vi "FFT_DAS Acq USB-Thermocouple.vi"(11 "Temp Channel":refnum<k21>) -> ()   [LabVIEW 2010]
doc: "I. Description:\nThis example demonstrates how to make temperature measurement using a thermocouple.\n\nII. Instructions for Running:\n1. Specify the Physical Channel where you have connected the thermocouple.\n2. Enter the Minimum and Maximum temperature values you expect to measure in degrees C. A smaller range will allow a more accurate measurement.\n3. Specify the type of thermocouple you are using.\n4. Thermocouple measurements require cold-junction compensation (CJC) to correctly scale them. Specify the source of your cold-junction compensation.\n5. If your CJC source is \"Internal\", skip the rest of steps.\n6. If your CJC source is \"Constant Value\", specify the value (usually room temperature) in degrees C.\n7. If your CJC source is \"Channel\", specify the CJC Channel name. \n\nIII. Block Diagram Steps:\n1. Create a Thermocouple (TC) temperature measurement channel.\n2. Call the Read VI to read one point of data.\n3. Call the Clear Task VI to clear the Task \n4. Use the popup dialog box to display an error if any.\n\nIV. I/O Connections Overview:\nConnect your thermocouple to the terminals corresponding to the Physical Channel I/O Control value."
uses:
  <vilib>/Utility/error.llb/DialogType.ctl
  <vilib>/Platform/TimedLoop/XDataNode/XDataNode.xnode
  <vilib>/Platform/TimedLoop/XDataNode/timing_clust.ctl
  <vilib>/Platform/TimedLoop/XDataNode/nitl_modes.ctl
  <vilib>/Platform/TimedLoop/XDataNode/wakeup.ctl
  <vilib>/DAQmx/read.llb/DAQmx Read (Analog DBL 1Chan 1Samp).vi
  <vilib>/daqmx/miscellaneous.llb/DAQmx Fill In Error Info.vi
  <vilib>/Platform/TimedLoop/XDataNode/XDNodeRunTimeDep.lvlib
panel:
  out "mSec":u32
  out "Loops":i32
  in  "stop":bool
  out "Measurement":cluster{"data":dbl, u32}(graph)
  out "Temperature":dbl(slide)=97.41100323624595 scale=0.0..100.0
  # "For instructions, select Help>>Show Context Help"
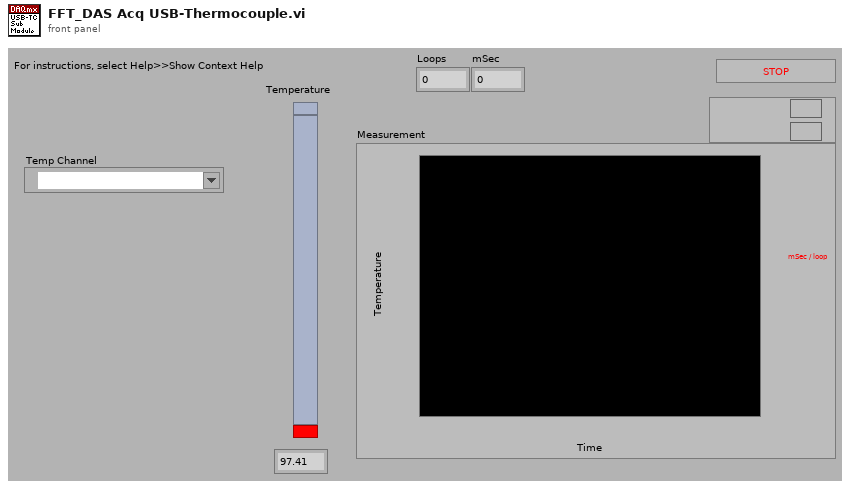
[diagram p1: front panel]
types:
  T1 = typedef "DialogType.ctl" = u16
  T2 = typedef "XDNodeRunTimeDep.lvlib/timing_clust.ctl" = cluster{"Expected End [f-1]":u64, "Actual End [f-1]":u64, "Finished Late? [f-1]":bool, "Expected End [i-1]":u64, "Actual End [i-1]":u64, "Finished Late? [i-1]":bool, "Expected Start [i]":u64, "Actual Start [i]":u64, "Expected Start [f]":u64, "Actual Start [f]":u64, "Source Name":string, "Structure Name":string, "Period":i64, "Deadline":i64, "Offset":i64, "Start":i64, "Priority":i32, "Timeout":i32, "Mode":T3, "Wakeup Reason":T4, "Error":errorcluster, "Source Type":string, "Secondary Source Type":string, "Global End Time":u64, "Global Start Time":u64, "Frame Duration":u64, "Iteration Duration":u64, "Assigned CPU":i32, "I/O Scan Engine Mode":u32}
  T3 = typedef "XDNodeRunTimeDep.lvlib/nitl_modes.ctl" = enum32{"No Change", "Process missed periods, maintain original phase", "Discard missed periods, maintain original phase", "Process missed periods, ignore original phase", "Discard missed periods, ignore original phase"}
  T4 = typedef "XDNodeRunTimeDep.lvlib/wakeup.ctl" = enum32{"Normal", "Aborted", "Asynchronous wakeup", "Timing source error", "Timed loop error", "Timeout"}
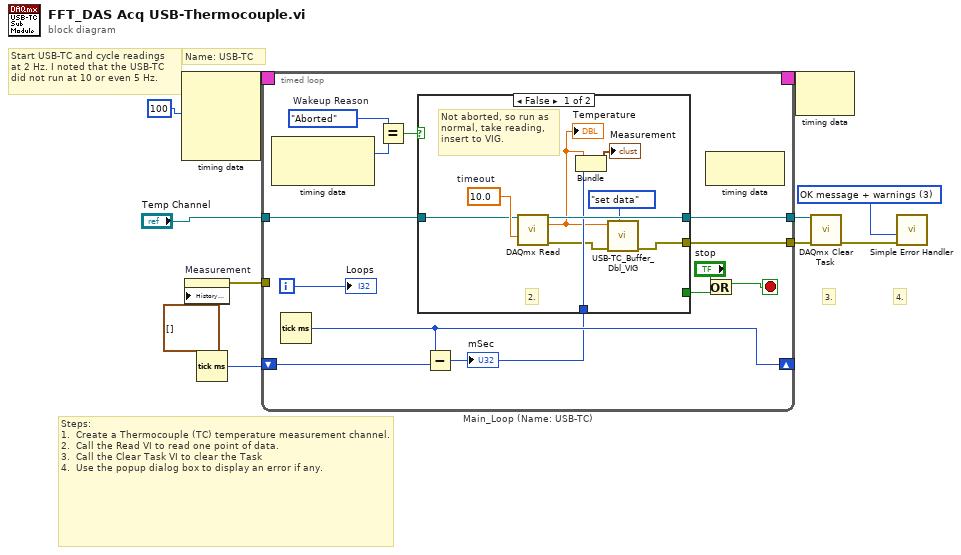
[diagram p0: block diagram]
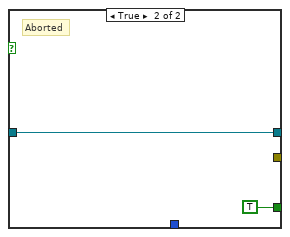
[diagram p2: hidden frame]
diagram:
  w11 = T1 3 items=["no dialog", "OK message", "continue or stop message", "OK message + warnings", "continue/stop + warnings"] ("type of dialog (OK msg:1)")
  # "Start USB-TC and cycle readings\nat 2 Hz. I noted that the USB-TC\ndid not run at 10 or even 5 Hz."
  # "Name: USB-TC"
  # "3."
  # "4."
  # "Steps: \n1.  Create a Thermocouple (TC) temperature measurement channel.\n2.  Call the Read VI to read one point of data.\n3.  Call the Clear Task VI to clear the Task  \n4.  Use the popup dialog box to display an error if any."
  n1 = node-c288(i64 100 ("Period")) -> (w7:T2)  [unwired: 3 in]
  n2 = property on="Measurement" class="WFChart (strict)"("History Data"=cluster{"data":dbl, u32}[] []) -> (error out=w4:errorcluster)  [unwired: 2 in, 1 out]
  n3 = Tick Count (ms)() -> (millisecond timer value=w3:u32)
  n4 = timed-loop "Main_Loop (Name: USB-TC)" {
    timing: w7 -> [_]
    timing-out: [_] -> w6
    tunnel: [w24] -> w10
    tunnel: [w23] -> w9
    tunnel: w4 -> [_]
    shift-right: [w19] -> _
    shift-left: w3 -> [w20]
    tunnel: "Temp Channel" -> [w12]
    i -> [w21]
    stop <- w14 stop-if-true
    w16 = wakeup."Aborted"  # Wakeup Reason
    n5 = node-c288() -> (w17:T4)  [unwired: 1 in, 1 out]
    n6 = Tick Count (ms)() -> (millisecond timer value=w19:u32)
    n7 = Equal?(x=w16, y=w17) -> (x = y?=w15:bool)
    n8 = Subtract(x=w19, y=w20) -> (x-y=w18:u32)
    "mSec" <- w18
    n9 = case shown="False" w15 {
      tunnel: [w32 w34] -> w24
      tunnel: [w27 _] -> w23
      tunnel: w18 -> [w31 _]
      tunnel: [_ TRUE] -> w13
      tunnel: w12 -> [w25 w34]
      frame False {
        w33 = 10.0  # timeout
        # "Not aborted, so run as\nnormal, take reading,\ninsert to VIG."
        # "2."
        n10 = call-poly <vilib>:"DAQmx Read.vi"("task/channels in"=w25, "timeout"=w33) -> ("task out"=w32:refnum<k21>, "data"=w29:dbl, "error out"=w28:errorcluster)  [unwired: 11 in]
        "Temperature" <- w29
        n11 = Bundle("data"=w29, w31) -> (→"Measurement":cluster{"data":dbl, u32})  [unwired: 1 in]
        n12 = call "USB-TC_Buffer_Dbl_VIG.vi"("Operation"=enum16{"get data", "set data", "initialize"}."set data", "error in"=w28, "Numeric"=w29) -> ("error out"=w27:errorcluster)  [unwired: 7 in, 1 out]
      }
      frame True {
        # "Aborted"
      }
    }
    n13 = node-c288() -> ()  [unwired: 1 in, 1 out]
    n14 = Or(x="stop", y=w13) -> (x .or. y?=w14:bool)
    "Loops" <- w21
  }
  n15 = node-c288(w6) -> ()  [unwired: 1 out]
  n16 = call <vilib>:"DAQmx Clear Task.vi"("task in"=w10, "error in"=w9) -> ("error out"=w8:errorcluster)  [unwired: 13 in]
  n17 = call <vilib>:"Simple Error Handler.vi"("type of dialog (OK msg:1)"=w11, "error in (no error)"=w8) -> ()  [unwired: 3 in, 5 out]
